vi "Point ToString.vi"(8 "error in (no error)":errorcluster caption="错误输入（无错误）", 11 "Point 输入":refnum<class "Point.lvclass"> caption="DNL_LabVIEW Object in") -> (0 "error out":errorcluster caption="错误输出", 2 "ToString":string, 3 "Point 输出":refnum<class "Point.lvclass"> caption="DNL_LabVIEW Object out")   [LabVIEW 2011, in "Point.lvclass"]
uses:
  Point.lvclass
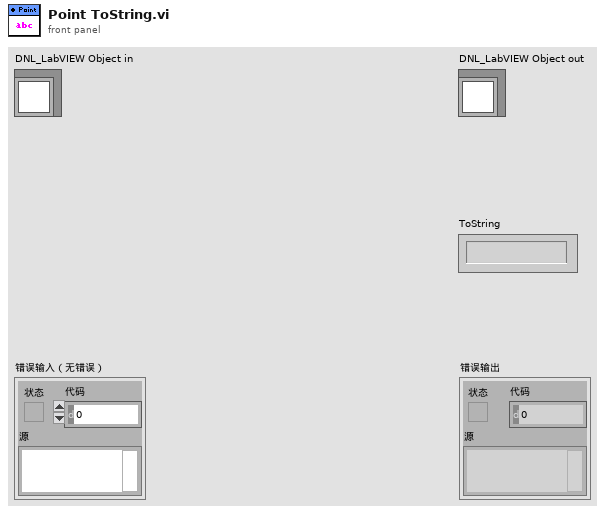
[diagram p1: front panel]
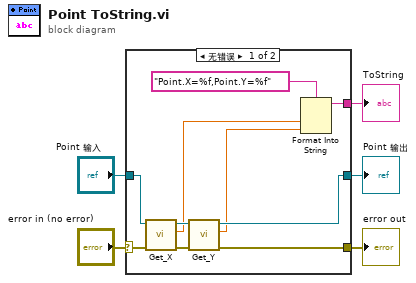
[diagram p0: block diagram]
diagram:
  n1 = case shown="无错误" "error in (no error)" {
    selector: "error in (no error)" -> [w9 w17]
    tunnel: [w6 w17] -> w4
    tunnel: [w13 w16] -> w2
    tunnel: "Point 输入" -> [w15 w16]
    tunnel: [w8 _] -> w1
    frame No Error {
      n2 = call "Get_X.vi"("error in (no error)"=w9, "Point输入"=w15) -> ("error out"=w7:errorcluster, "X"=w11:dbl, "Point输出"=w14:refnum<class "Point.lvclass">)  [unwired: 7 in]
      n3 = call "Get_Y.vi"("error in (no error)"=w7, "Point输入"=w14) -> ("error out"=w6:errorcluster, "Y"=w10:dbl, "Point输出"=w13:refnum<class "Point.lvclass">)  [unwired: 7 in]
      n4 = Format Into String(format string="Point.X=%f,Point.Y=%f" ("格式字符串"), w11, w10) -> (resulting string=w8:string)  [unwired: 2 in, 1 out]
    }
    frame Error {
    }
  }
  "error out" <- w4
  "Point 输出" <- w2
  "ToString" <- w1
